vi "DXF Parser Example.vi"() -> ()   [LabVIEW 2014] (continued)
11.18013928322898, 11.18117027556996, 11.17359484963523, 11.15262768649381, 11.14335070901023, 11.15018599860088, 11.15834094338523, 11.16672704906302, 11.17329406838523, 11.17824411545825], "Y"=[20.98014850304497, 20.88142199659544, 20.8664495284356, 20.85565280770329, 20.84463092491997, 20.83907500299597, 20.8250481612481, 20.80254284864494, 20.7125569503106, 20.67461464507574, 20.52228912804497, 20.44466678394849, 20.42625372765436, 20.42100200920926, 20.43302350304497, 20.44434583600054, 20.46070904991998, 20.47601794878094, 20.53753204796685, 20.58196147597581, 20.63129889366998, 20.65967497965404, 20.67555157921685, 20.68044962822679, 20.67064850304498, 20.66332078797728, 20.6709133956231, 20.68087818504184, 20.73649225304498, 20.86343461614308, 20.99463678429498, 21.06952477081995, 21.08349029991997, 21.08156492670809, 21.06481061241998, 21.04668636734289]}, {"X"=[10.82500109963523, 10.93621457789177, 10.95515344338523, 10.98582849687807, 11.04142297463523, 11.12367529376433, 11.30589172463523, 11.36794763097458, 11.42676199441062, 11.4210015232437, 11.35689718728171, 11.27560415844139, 11.12739489846336, 11.09426758470566, 11.07404797463523, 11.06603194388106, 11.05326672463523, 11.0334041057101, 11.01301672463523, 10.99396770383149, 10.97364416604148, 10.96196081379431, 10.94342688088523, 10.92879282103845, 10.90983343606101, 10.89307016172453, 10.86717297463523, 10.84578575884946, 10.82242492776023, 10.80590475867271, 10.79206164651023, 10.77926402785334, 10.76627673440085, 10.75169283177581, 10.72401672463523, 10.60267738925845, 10.54485165505515, 10.52463742420986, 10.5316854258071, 10.55244731181157, 10.62357727151023, 10.68258955070349, 10.78801672463523, 10.80648243729615], "Y"=[20.28853912804497, 20.24982826384868, 20.24739264366998, 20.25375449108233, 20.27082037804498, 20.26584408186534, 20.17494537804497, 20.12085267949265, 19.99075012658013, 19.86928774959328, 19.69147217247857, 19.55200990301619, 19.36537164757623, 19.33193741557578, 19.32913287804497, 19.33558642850907, 19.35389850304497, 19.39459118286949, 19.43502350304497, 19.45823820369493, 19.46105743859185, 19.45121417952689, 19.42977936241998, 19.42113724850345, 19.42390689537896, 19.44093499389652, 19.47690631554498, 19.49414486329342, 19.49214362023248, 19.46941267843274, 19.44495904991998, 19.43723225611936, 19.43934015343561, 19.45321929808048, 19.50302350304498, 19.80177938242652, 20.00464404747857, 20.15408196243347, 20.23704840538873, 20.28697934578785, 20.33491022179498, 20.33448612687505, 20.30302350304498, 20.29571371474227]}, {"X"=[9.835016724635228, 9.813012981431298, 9.814091675807106, 9.82240079736692, 9.83498352151023, 9.875232494428754, 9.95642883401023, 10.04861961421355, 10.05364172463523, 10.04033287102509, 10.01904797463523, 9.969425173364687, 9.94311047463523, 9.936361381348698, 9.914891724635229, 9.861860989545756], "Y"=[20.61602350304497, 20.68391098860619, 20.69438849327935, 20.69602531737148, 20.68355865929498, 20.63453822835508, 20.52379303429498, 20.37847042523036, 20.36102350304498, 20.34922456611368, 20.35234772179498, 20.35477554304546, 20.35973053429498, 20.36564430530411, 20.40764850304497, 20.54266898942641]}, {"X"=[9.20801672463523, 8.944247230825384, 8.905942505885228, 8.898246311277997, 8.89961633401023, 8.919412093509825, 9.02665734963523, 9.121851033395467, 9.21732531838523, 9.328365326043858, 9.425122193385228, 9.482290230673826, 9.49663586526023, 9.498494385396762, 9.46239172463523, 9.438341281381721, 9.42202453713523, 9.388701189537835, 9.28651672463523, 9.251553198491818], "Y"=[19.16852350304498, 19.23148256953707, 19.24623444054498, 19.25230813252803, 19.26458404991997, 19.27166194859355, 19.26822662804498, 19.25634879079069, 19.24699029991998, 19.24432871652031, 19.24976373741998, 19.25704432704663, 19.25477545616998, 19.24033414513041, 19.20014850304498, 19.16836303487901, 19.15741217491998, 19.15241091539771, 19.15628912804497, 19.16048311016624]}, {"X"=[10.24289172463523, 10.11694505397632, 9.99373547463523, 9.859689792691393, 9.71792541604148, 9.626855452734858, 9.61231115822898, 9.634862241259896, 9.69618469338523, 9.753346696259383, 9.77818274026023, 9.781551565281118, 9.80466711526023, 9.848778436907564, 9.872555787135228, 9.900119708063901, 9.904704224635228, 9.907885509886404, 9.92395422463523, 9.97817736082229, 10.03476165871726, 10.1530175867297, 10.25825158791648, 10.36984261473868, 10.57590393166648, 10.64091672068687, 10.64319522194968, 10.62389268310771, 10.60064172463523, 10.55928217749618, 10.52616320901023, 10.50421478369177, 10.51479992776023, 10.54162040674538, 10.54201672463523, 10.52859188259705, 10.47910461526023, 10.40767155381768], "Y"=[19.31714850304498, 19.34980077721107, 19.37113678429498, 19.39781047645481, 19.46403394005669, 19.56658476095363, 19.64561529991998, 19.69663770909627, 19.75158600304498, 19.78227090552736, 19.80704962609185, 19.81839491403495, 19.85943439171685, 19.88607796737461, 19.90038287804497, 19.95092246032508, 20.00639850304497, 20.04328657628024, 20.08208600304497, 20.12787903093948, 20.14135037682427, 20.10910235221808, 20.03463165734185, 19.91685712865697, 19.58889142296685, 19.42834574533098, 19.40343863366022, 19.38798992555383, 19.39189850304498, 19.40283782254223, 19.40288483116998, 19.36885028040541, 19.34031256554497, 19.29867528148893, 19.25902350304498, 19.25053447166477, 19.25090240929498, 19.26600363647589]}, {"X"=[10.68401672463523, 10.74012237131718, 10.75910461526023, 10.78685678147583, 10.80401672463523, 10.82804589112411, 10.84539172463523, 10.86110803636856, 10.87780578713523, 10.8961034555522, 10.91401672463523, 10.93172250790367, 10.95404211526023, 10.97550491556371, 10.98953234963523, 11.00081533108493, 11.01301672463523, 11.02346382950975, 11.03273547463523, 11.047234612202, 11.08867297463523, 11.16402669168347, 11.25270446877585, 11.32391502338663, 11.32467727761374, 11.29810613643917, 11.25501672463523, 11.19144843530136, 11.11601672463523, 11.03790628411923, 10.99579211526023, 10.92089396391901, 10.84599133401023, 10.80929775115956, 10.77398352151023, 10.73887799959298, 10.67331359963523, 10.58539050059224, 10.48302307229148, 10.47479498249245, 10.52197326760398, 10.56224666194883, 10.64401672463523, 10.67394228004621], "Y"=[18.62302350304498, 18.71026723165782, 18.72816022179498, 18.72358145208433, 18.70302350304497, 18.67244711692641, 18.66144537804497, 18.66716524286067, 18.69496686241997, 18.72485879182673, 18.73302350304498, 18.72362058940694, 18.69322662804498, 18.66210308142931, 18.65427350304497, 18.6603997266632, 18.68502350304497, 18.69932335761112, 18.70250787804497, 18.6966818381585, 18.65535162804498, 18.56200172164521, 18.42335113976373, 18.2260086995535, 18.08534302208795, 18.00954917862288, 17.95002350304498, 17.91192370964248, 17.90902350304498, 17.93645196298704, 17.95106451866997, 17.95021554690091, 17.94999225304498, 17.95792919948559, 17.96049225304498, 17.95648896958128, 17.95444537804498, 17.98025752374457, 18.09835333702935, 18.23983425015326, 18.3751965987481, 18.4465457070874, 18.56702350304498, 18.60866692724437]}, {"X"=[10.50451672463523, 10.35965101499587, 10.28022961526023, 10.20099424712611, 10.06878234963523, 9.979258102610848, 9.92201672463523, 9.822373957859854, 9.79490734963523, 9.773496750579755, 9.762407349635227, 9.759705379466485, 9.74759484963523, 9.712991837432277, 9.675605835963356, 9.658667758617668, 9.653126587916478, 9.669767703809237, 9.749385682154761, 9.837103551257357, 9.98901672463523, 10.20451058797383, 10.4287332773696, 10.5161757838527, 10.53104422097312, 10.52862450654114, 10.5077733164321, 10.49974346399592, 10.51214172463523, 10.55355176019783, 10.57735022072898, 10.59148730792228, 10.59406311135398, 10.58311051141433, 10.55586047463523, 10.54685159688748, 10.56309484963523, 10.59729171826548, 10.63093664651023, 10.64942943125121, 10.65709387307273, 10.65309560679298, 10.59726672463523, 10.56222553284077], "Y"=[18.58827350304497, 18.44051210567195, 18.37979889366998, 18.34362849488037, 18.35060162804498, 18.41503912519286, 18.48502350304497, 18.56567203231591, 18.58229889366998, 18.60679950859787, 18.63886505577935, 18.67333422575752, 18.73635162804498, 18.79381753309326, 18.8495130049981, 18.89515649500408, 18.99000177452935, 19.04700715265889, 19.15149493859185, 19.19994386141475, 19.22577350304498, 19.20769398530136, 19.14922076866997, 19.11499769895063, 19.10110919640434, 19.08276280219706, 19.05605670616998, 19.02335085910856, 18.99739850304498, 18.97469977658506, 18.96567438195123, 18.95271476440298, 18.93918024132623, 18.91665839725065, 18.87905475304498, 18.84876137687651, 18.82771100304497, 18.82846017422566, 18.83462506554498, 18.8309681845875, 18.82049518273248, 18.79137589972013, 18.70002350304497, 18.65528873723261]}, {"X"=[9.259016724635229, 9.284438152560849, 9.30617102151023, 9.325045924029101, 9.35334484963523, 9.390172713231875, 9.410139527369605, 9.423201850363327, 9.42801672463523, 9.433389281615685, 9.461643677760229, 9.49669664272346, 9.65598059182273, 9.828448626461181, 9.871874024439917, 9.884075818374544, 9.851667115260229, 9.810245549910132, 9.78822961526023, 9.770075311968753, 9.763688599635229, 9.719695399140862, 9.645087037135228, 9.616184625836087, 9.57301672463523, 9.531285724263773, 9.480266724635229, 9.442385716108191, 9.40859533791648, 9.34905455150492, 9.29377453713523, 9.261559295509933, 9.251797974635227, 9.255261788513716], "Y"=[17.27502350304497, 17.3989150571542, 17.42248834679498, 17.42225229866207, 17.40588287804498, 17.38250979377885, 17.3794397628106, 17.39241158135267, 17.42402350304497, 17.45709985458265, 17.48496686241997, 17.48400744474597, 17.41326276085747, 17.27047925709038, 17.20210663292779, 17.13598125025857, 17.07454498741998, 17.05212853552449, 17.03953912804498, 17.00599586091519, 16.95664850304497, 16.86859026823781, 16.83641901085748, 16.83899705383438, 16.85102350304497, 16.8645947312819, 16.87039850304497, 16.86957546268594, 16.8732268721856, 16.89580407830343, 16.95026446984185, 17.03559318296808, 17.17822858116998, 17.22663689773219]}, {"X"=[9.177358521510229, 9.155557191806656, 9.123306519557106, 9.059870486080227, 8.914430054713355, 8.89524659336215, 8.87901672463523, 8.865265258733013, 8.84989172463523, 8.830635231299674, 8.77801672463523, 8.743497985734978, 8.72422766213523, 8.701541629033906, 8.675696412135228, 8.640549448230669, 8.580195679713356, 8.545347138624997, 8.557016724635229, 8.600554787551074, 8.71768762307273, 8.794374603599026, 8.956251099635228, 9.028391048464346, 9.053501099635229, 9.062658966552227, 9.05195422463523, 9.050780068305063, 9.08037414651023, 9.104437394193608, 9.13889172463523, 9.158060032232408, 9.16846984963523, 9.175380127259155, 9.179016724635229, 9.178627056786976], "Y"=[17.37569342491998, 17.20907862120462, 17.11962384484185, 17.04408092214745, 17.03702447960747, 17.05130541721442, 17.06802350304498, 17.0868001269925, 17.10427350304498, 17.11632621131707, 17.13602350304497, 17.15106016197962, 17.16690826866997, 17.19562785308022, 17.22154108116998, 17.24209312184824, 17.28755768273248, 17.38531674467066, 17.44902350304498, 17.53986156023845, 17.63739850304497, 17.65766041416526, 17.66458014366997, 17.6524906547778, 17.63670904991998, 17.59973733331313, 17.55207037804498, 17.51830975572069, 17.48165631554497, 17.47979984392449, 17.48552350304498, 17.48439563989126, 17.47771100304497, 17.46280489151818, 17.42002350304498, 17.40399698046572]}, {"X"=[9.58201672463523, 9.718586369711499, 9.81489172463523, 9.913593397005116, 9.942165650416479, 9.990285265836146, 10.07101672463523, 10.10544479287385, 10.12336438088523, 10.13189418981126, 10.14386047463523, 10.17863835097603, 10.20019275002585, 10.2103917572688, 10.17278039651023, 10.14922321595798, 10.12872448830711, 10.11731075811736, 10.11188586526023, 10.10301528384602, 10.06746594338523, 9.982111102478981, 9.848467896510229, 9.61799413574987, 9.542562378932104, 9.500142079559064, 9.495905640650854, 9.50462367128683, 9.53768859963523, 9.55703054613882, 9.564126099635228, 9.549810785431214, 9.516563599635228, 9.5062970156662, 9.508546021510229, 9.516146243542138, 9.55001672463523, 9.566021223979272], "Y"=[17.81202350304497, 17.89320802015305, 17.96024225304497, 18.03823123631414, 18.0517542159356, 18.04699569893543, 17.98902350304498, 17.9387298380442, 17.88898639366997, 17.84222685092788, 17.79622662804498, 17.73241574629938, 17.69973907921685, 17.61734665767417, 17.54417389366997, 17.51654450248837, 17.48657574913872, 17.44891663779161, 17.40605865929498, 17.36627570595532, 17.32961139366998, 17.32867352863639, 17.38284381554498, 17.50502422388584, 17.55436237023248, 17.59431901533173, 17.61123248741998, 17.62297829224688, 17.64014850304498, 17.65516419816567, 17.67800787804498, 17.70667382389182, 17.74057037804497, 17.75630562484394, 17.77015045616997, 17.77619988451326, 17.79502350304498, 17.80351503369148]}, {"X"=[9.25395617776023, 9.212900929016081, 9.206258179713355, 9.30399186824802, 9.398115479518042, 9.510439254581149, 9.563090577174293, 9.592709077929188, 9.652422974635229, 9.71538025472824, 9.77523547463523, 9.81130043365502, 9.758600953150856, 9.696964288823299, 9.55001672463523, 9.514973341681957, 9.470607544947729, 9.447493297004641, 9.421610718775854, 9.392664253773818, 9.365967896510229, 9.343791936197393, 9.31236242776023, 9.295306096948856], "Y"=[18.02978522179497, 18.17720205374536, 18.31080621788873, 18.50033405139931, 18.55152185509576, 18.54378836856382, 18.50947717736138, 18.47505565553923, 18.41553912804498, 18.37813547969026, 18.33594537804498, 18.19010951987187, 18.08870709679498, 18.01574858953538, 17.90002350304497, 17.88221302417681, 17.88527154991998, 17.90523022818386, 17.92143854210747, 17.91665446934491, 17.89940631554497, 17.88909834090587, 17.89826569054497, 17.92492467990929]}, {"X"=[8.86889172463523, 8.794731912480541, 8.720376099635232, 8.582683234473333, 8.52926721291648, 8.478366715977069, 8.43356750588523, 8.431154458837211, 8.41948547463523, 8.399043311311633, 8.39344787697898, 8.408622935671136, 8.50576672463523, 8.620061588476338, 8.64873498635398, 8.706484922535877, 8.75851672463523, 8.804169174965056, 8.87059533791648, 8.945927693026155, 9.009671021510231, 9.057917915094244, 9.16279016213523, 9.179562211198691, 9.16620129494773, 9.141071794759112, 9.09346203713523, 9.036766469433463, 9.013699585963355, 9.006007106847358, 9.007788209010231, 8.992703275614803, 8.96301672463523, 8.94402103827468], "Y"=[17.80139850304498, 17.81771674173077, 17.83311725304497, 17.8590678143351, 17.8750686690606, 17.90486798168387, 17.98220514366998, 18.02426162274768, 18.10158600304498, 18.15794549038706, 18.20104303429497, 18.23152521078015, 18.28314850304498, 18.29210958646645, 18.29239313195123, 18.30987173578658, 18.33952350304498, 18.36252047909635, 18.37057574913872, 18.33422643327366, 18.26136334679497, 18.18035763667963, 17.95668756554497, 17.90587433883467, 17.87969440148247, 17.87434097113529, 17.87245319054497, 17.86777805640396, 17.85703082726372, 17.83198235895912, 17.80583990929497, 17.78650379130455, 17.78302350304498, 17.78576261640105]}, {"X"=[8.29959484963523, 8.234575376623265, 8.201108521510228, 8.179274771242051, 8.171501099635229, 8.160625773780422, 8.14801672463523, 8.127030425220221, 8.085385865260232, 8.00833164299031, 7.936890503932103, 7.883817068850907, 7.768794068385229, 7.684656425435913, 7.617219849635229, 7.594526011939912, 7.594216950465308, 7.601898374674585, 7.66045227151023, 7.740852159644955, 7.784766724635229, 7.802722650629203, 7.812016724635229, 7.825181934403298, 7.841378296900854, 7.863167302826963, 7.90527258401023, 7.990601840909938, 8.177010865260229, 8.247494025321167, 8.30601672463523, 8.336969520039876, 8.356516724635231, 8.361600633551657, 8.347391724635228, 8.323867737641628], "Y"=[17.23783600304498, 17.18597113973961, 17.15521881554498, 17.13279643203634, 17.13069537804498, 17.14034307762222, 17.16402350304498, 17.17520645229135, 17.17142389366997, 17.15864170150324, 17.15404181359185, 17.15944392699114, 17.18292779991998, 17.20810996376595, 17.23808600304498, 17.2545698859186, 17.26033990929498, 17.26402062730205, 17.26003912804498, 17.24478521170542, 17.24089850304497, 17.24454385826968, 17.25102350304498, 17.2680652825209, 17.28225763390435, 17.28487485313375, 17.27304889366998, 17.25416114244922, 17.25641412804498, 17.27318089168439, 17.29902350304497, 17.31351822095487, 17.31139850304498, 17.29384452637549, 17.27452350304497, 17.25569191484265]}]
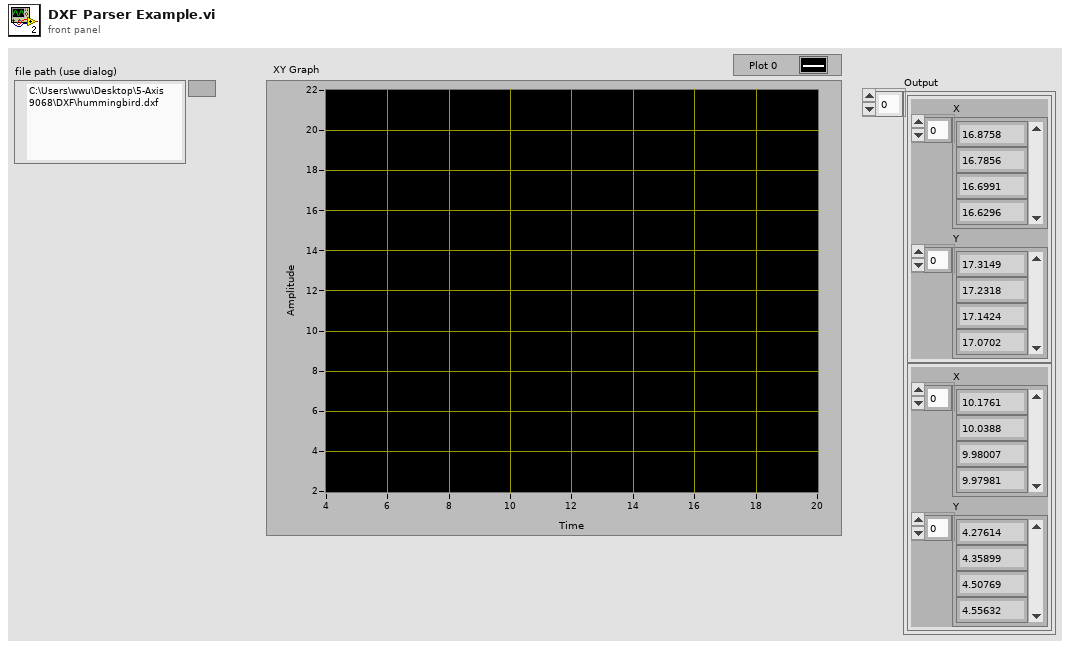
[diagram p1: front panel]
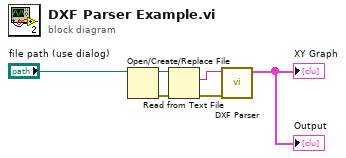
[diagram p0: block diagram]
diagram:
  n1 = Open/Create/Replace File(file path (use dialog)="file path (use dialog)") -> (refnum out=w6:refnum<file>, error out=w5:errorcluster)  [unwired: 5 in, 1 out]
  n2 = Read from Text File(file (use dialog)=w6, error in=w5) -> (text=w3:string, error out=w4:errorcluster)  [unwired: 2 in, 2 out]
  n3 = call "DXF Parser.vi"("error in (no error)"=w4, "String in"=w3) -> ("Output"=→"XY Graph" →"Output":cluster{"X":dbl[], "Y":dbl[]}[])  [unwired: 8 in, 1 out]
